vi "Calc Inputs.vi"(8 "error in (no error)":errorcluster, 11 "Calculation in":refnum<class "Calculation.lvclass">) -> (0 "error out":errorcluster, 2 "Inputs":string[](array[string]))   [LabVIEW 2020, in "VolatusCalcs.lvlib" / "Calculation.lvclass"]
uses:
  Calculation.lvclass
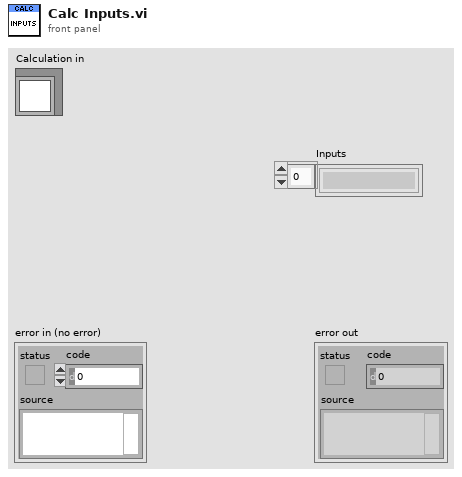
[diagram p1: front panel]
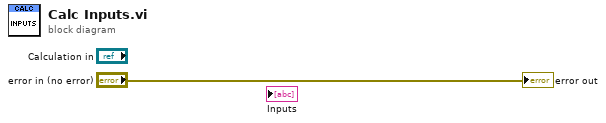
[diagram p0: block diagram]
diagram:
  "error out" <- "error in (no error)"
